vi "VCS Digital Input Configuration.vi"(8 "error in (no error)":errorcluster, 10 "input configuration":T1={"digitalInputNumber"=1, "configuration"=15, "mask"=1, "polarity"=0, "executionMask"=1} {"executionMask" items=["Disabled", "Enabled"]; "polarity" items=["HighActive", "LowActive"]; "mask" items=["Disabled", "Enabled"]; "configuration" items=["Negative Limit Switch"=0, "Positive Limit Switch"=1, "Home Switch"=2, "Position Marker"=3, "Enable"=4, "Quick Stop"=5, "General Purpose A"=15, "General Purpose B"=14, "General Purpose C"=13, "General Purpose D"=12, "General Purpose E"=11, "General Purpose F"=10, "General Purpose G"=9, "General Purpose H"=8]}, 11 "axis in":cluster{"keyHandle":u32, "nodeId":u16}={"keyHandle"=0, "nodeId"=1}) -> (0 "error out":errorcluster, 3 "axis out":cluster{"keyHandle":u32, "nodeId":u16}={"keyHandle"=0, "nodeId"=1})   [LabVIEW 2017, in "maxonEPOS.lvlib"]
doc: "<B>VCS Digital Input Configuration</B> sets parameter for one digital input."
uses:
  Examples/maxonEPOS.lvlib
  Resources/EposCmd.dll
  SSI_Tool/InstrumentsInterfaces/Motordriver/maxon EPOS/Resources/EposCmd64.dll
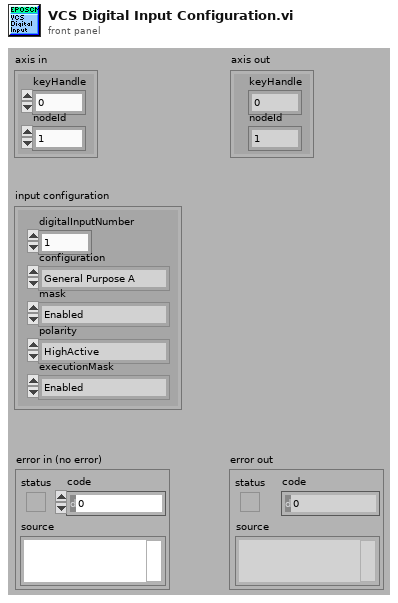
[diagram p1: front panel]
types:
  T1 = cluster{"digitalInputNumber":u16, "configuration":u16, "mask":i32, "polarity":i32, "executionMask":i32}
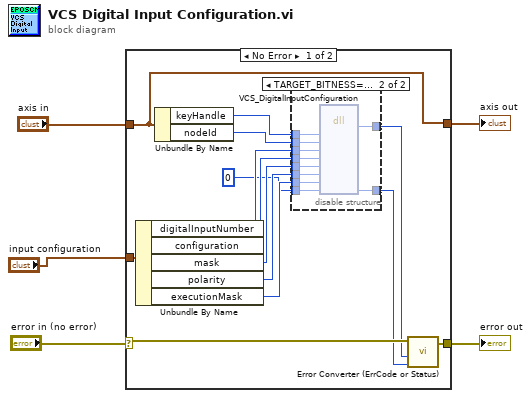
[diagram p0: block diagram]
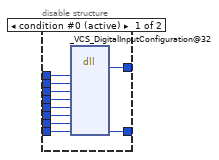
[diagram p2: hidden frame]
diagram:
  n1 = case shown="No Error" "error in (no error)" {
    selector: "error in (no error)" -> [w8 w41]
    tunnel: [w9 w41] -> w4
    tunnel: "axis in" -> [w11 w40]
    tunnel: "input configuration" -> [w17 _]
    tunnel: [w11 w40] -> w1
    frame No Error {
      n2 = Unbundle By Name(w17) -> ("digitalInputNumber"=w16:u16, "configuration"=w15:u16, "mask"=w14:i32, "polarity"=w13:i32, "executionMask"=w12:i32)
      n3 = Unbundle By Name(w11) -> ("keyHandle"=w19:u32, "nodeId"=w18:u16)
      n4 = disable-structure shown="TARGET_BITNESS==64" {
        disable-tunnel: w19 -> [w29 w39]
        disable-tunnel: w18 -> [w28 w38]
        disable-tunnel: w16 -> [w27 w37]
        disable-tunnel: w15 -> [w26 w36]
        disable-tunnel: w14 -> [w25 w35]
        disable-tunnel: w13 -> [w24 w34]
        disable-tunnel: w12 -> [w23 w33]
        disable-tunnel: u32 0 ("pErrorCode") -> [w22 w32]
        disable-tunnel: [w21 w31] -> w7
        disable-tunnel: [w20 w30] -> w6
        frame condition #0 (active) {
          n5 = dll-call lib="C:/workspace/project/scancon/sw/SSI_Tool/InstrumentsInterfaces/Motordriver/maxon EPOS/Resources/EposCmd.*" fn="_VCS_DigitalInputConfiguration@32"("KeyHandle"=w29, "NodeId"=w28, "DigInputNb"=w27, "Configuration"=w26, "Mask"=w25, "Polarity"=w24, "ExecutionMask"=w23, "pErrorCode"=w22) -> (w21:i32, "pErrorCode"=w20:u32)  [unwired: 10 in, 2 out]
        }
        frame condition #1 {
          n6 = dll-call lib="C:/Sources/LabView/maxon EPOS/Resources/EposCmd64.*" fn="VCS_DigitalInputConfiguration" ("EposCmd.dll:_VCS_DigitalInputConfiguration@32")("KeyHandle"=w39, "NodeId"=w38, "DigInputNb"=w37, "Configuration"=w36, "Mask"=w35, "Polarity"=w34, "ExecutionMask"=w33, "pErrorCode"=w32) -> ("Rückgabetyp"=w31:i32, "pErrorCode"=w30:u32)  [unwired: 10 in, 2 out]
        }
      }
      n7 = call "Error Converter (ErrCode or Status).vi"("error code"=w6, "return type"=w7, "error in (no error)"=w8) -> ("error out"=w9:errorcluster)  [unwired: 7 in]
    }
    frame Error {
    }
  }
  "error out" <- w4
  "axis out" <- w1
